vi "FastMap - Visualize.vi"(11 "fast map in":refnum<data-value>) -> (3 "fast map out":refnum<data-value>)   [LabVIEW 2015, in "DS Square.lvlib"]
uses:
  DS Square.lvlib
  Square State Fast.ctl
  Fast Map.ctl
panel:
  out "Battlefield":i8[][](graph)
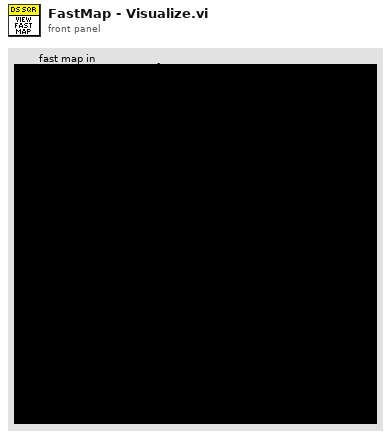
[diagram p1: front panel]
types:
  T1 = typedef "DS Square.lvlib/Square State Fast.ctl" = enum8{"Unknown", "Empty", "Occupied - Active", "Occupied - Cool Down", "Attacked", "Enemy", "Enemy Wall"}
  T2 = typedef "DS Square.lvlib/Fast Map.ctl" = cluster{"state":T1[][], "updated":i32[][]}
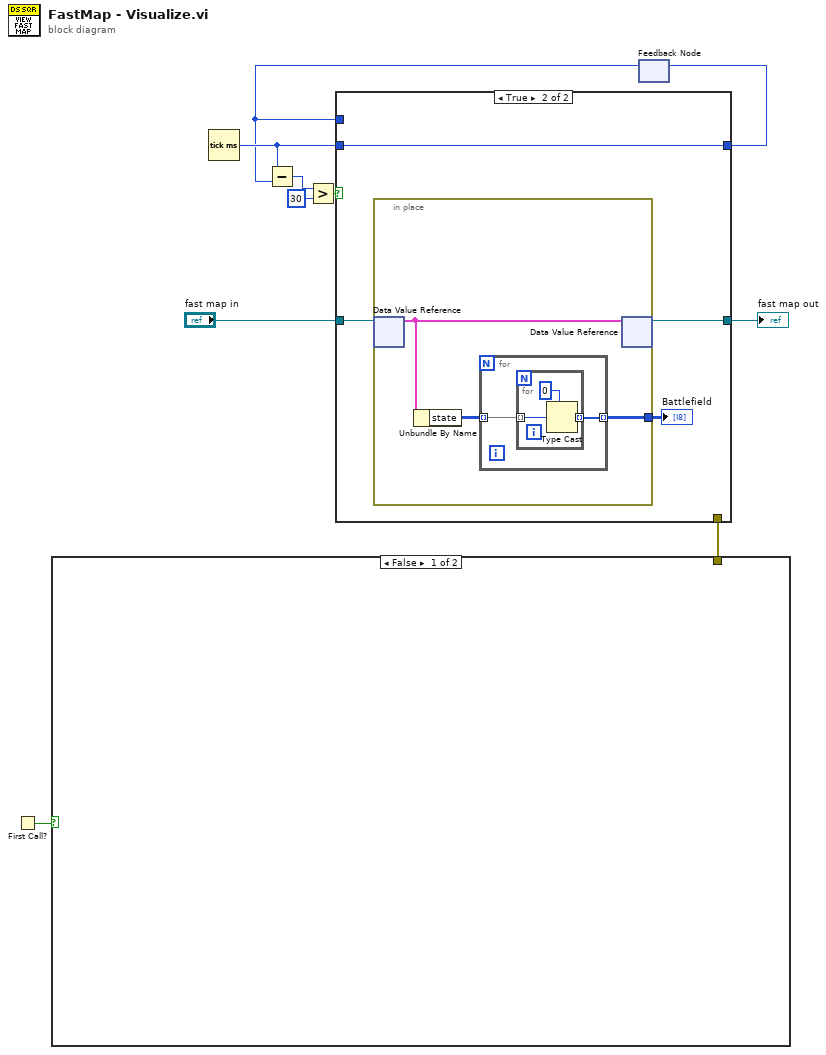
[diagram p0: block diagram]
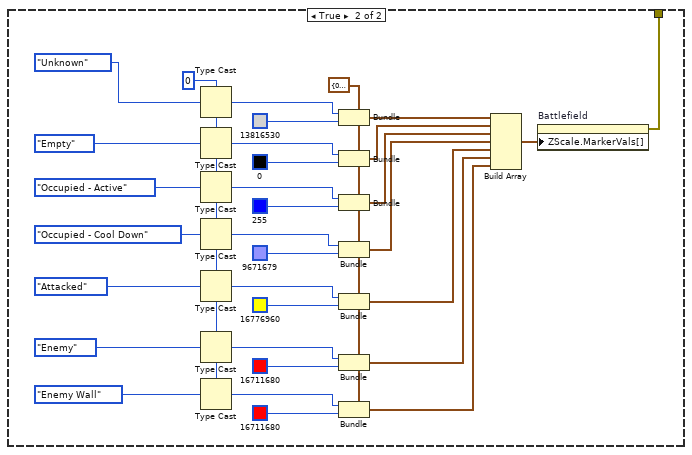
[diagram p3: hidden frame]
diagram:
  n1 = First Call?() -> (First Call?: T/F=w4:bool)
  n2 = case shown="False" w4 {
    tunnel: [_ w42] -> w8
    frame False {
    }
    frame True {
      w23 = i8 0 ("y")
      w26 = cluster{dbl, u32} {0.0, 0}
      n3 = Type Cast(type=w23, x=Square_State_Fast."Unknown" ("square state")) -> (*(type *) &x=w25:i8)
      n4 = Type Cast(type=w23, x=Square_State_Fast."Empty" ("square state")) -> (*(type *) &x=w24:i8)
      n5 = Type Cast(type=w23, x=Square_State_Fast."Occupied - Active" ("square state")) -> (*(type *) &x=w22:i8)
      n6 = Type Cast(type=w23, x=Square_State_Fast."Occupied - Cool Down" ("square state")) -> (*(type *) &x=w21:i8)
      n7 = Type Cast(type=w23, x=Square_State_Fast."Attacked" ("square state")) -> (*(type *) &x=w20:i8)
      n8 = Type Cast(type=w23, x=Square_State_Fast."Enemy" ("square state")) -> (*(type *) &x=w19:i8)
      n9 = Type Cast(type=w23, x=Square_State_Fast."Enemy Wall" ("square state")) -> (*(type *) &x=w18:i8)
      n10 = Bundle(cluster=w26, w25, u32 13816530) -> (w38:cluster{dbl, u32})
      n11 = Bundle(cluster=w26, w24, u32 0) -> (w37:cluster{dbl, u32})
      n12 = Bundle(cluster=w26, w22, u32 255) -> (w35:cluster{dbl, u32})
      n13 = Bundle(cluster=w26, w21, u32 9671679) -> (w30:cluster{dbl, u32})
      n14 = Bundle(cluster=w26, w20, u32 16776960) -> (w29:cluster{dbl, u32})
      n15 = Bundle(cluster=w26, w19, u32 16711680) -> (w28:cluster{dbl, u32})
      n16 = Bundle(cluster=w26, w18, u32 16711680) -> (w27:cluster{dbl, u32})
      n17 = Build Array(w38, w37, w35, w30, w29, w28, w27) -> (w41:cluster{dbl, u32}[])
      n18 = property on="Battlefield" class="IntGraph (strict)"("ZScale.MarkerVals[]"=w41) -> (error out=w42:errorcluster)  [unwired: 2 in, 1 out]
    }
  }
  n19 = Tick Count (ms)() -> (millisecond timer value=w2:u32)
  n20 = feedback #1() -> (w1:u32)  [unwired: 1 in]
  n21 = Subtract(x=w2, y=w1) -> (x-y=w7:u32)
  n22 = Greater?(x=w7, y=u32 30) -> (0:w5:bool)
  n23 = case shown="True" w5 {
    tunnel: "fast map in" -> [w44 w48]
    tunnel: [w44 w47] -> w9
    tunnel: w8 -> [_ _]
    tunnel: [w43 w46] -> w3
    tunnel: w2 -> [_ w46]
    tunnel: w1 -> [w43 _]
    frame False {
    }
    frame True {
      n24 = in-place {
        in-place-border: [w49] -> w45
        n25 = in-place-dvr #2(w48) -> (w51:T2)  [unwired: 1 out]
        n26 = Unbundle By Name(w51) -> ("state"=w50:T1[][])
        n27 = for {
          tunnel: w50 -> [w53] mode=indexing
          tunnel: [w52] -> w49 mode=indexing
          n28 = for {
            tunnel: w53 -> [w55] mode=indexing
            tunnel: [w54] -> w52 mode=indexing
            n29 = Type Cast(type=i8 0 ("y"), x=w55) -> (*(type *) &x=w54:i8)
          }
        }
        n30 = in-place-dvr #2(w51) -> (w47:refnum<data-value>)  [unwired: 1 out]
      }
      "Battlefield" <- w45
    }
  }
  "fast map out" <- w9
  n31 = feedback-in #1(w3) -> ()
